vi "ColorScores.vi"() -> ()   [LabVIEW 2022 SP3]
uses:
  <vilib>/Utility/file.llb/Read Delimited Spreadsheet (DBL).vi
  <vilib>/Analysis/NI_AALBase.lvlib
panel:
  out "Array Constant":u8[](array[numeric])
  out "min score":sgl
  out "max score":sgl
  in  "Save to BMP":bool
  in  "Listbox":i32[](listbox)=[0]
  in  "Use Selected Files":bool
  in  "Color Table":u32[](array[colorbox])=[0, 0, 65793, 131586, 197379, 263172, 328965, 394758, 460551, 526344, 592137, 657930, 723723, 789516, 855309, 921102, 986895, 1052688, 1118481, 1184274, 1250067, 1315860, 1381653, 1447446, 1513239, 1579032, 1644825, 1710618, 1776411, 1842204, 1907997, 1973790, 2039583, 2105376, 2171169, 2236962, 2302755, 2368548, 2434341, 2500134, 2565927, 2631720, 2697513, 2763306, 2829099, 2894892, 2960685, 3026478, 3092271, 3158064, 3223857, 3289650, 3355443, 3421236, 3487029, 3552822, 3618615, 3684408, 3750201, 3815994, 3881787, 3947580, 4013373, 4079166, 4144959, 4210752, 4276545, 4342338, 4408131, 4473924, 4539717, 4605510, 4671303, 4737096, 4802889, 4868682, 4934475, 5000268, 5066061, 5131854, 5197647, 5263440, 5329233, 5395026, 5460819, 5526612, 5592405, 5658198, 5723991, 5789784, 5855577, 5921370, 5987163, 6052956, 6118749, 6184542, 6250335, 6316128, 6381921, 6447714, 6513507, 6579300, 6645093, 6710886, 6776679, 6842472, 6908265, 6974058, 7039851, 7105644, 7171437, 7237230, 7303023, 7368816, 7434609, 7500402, 7566195, 7631988, 7697781, 7763574, 7829367, 7895160, 7960953, 8026746, 8092539, 8158332, 8224125, 8289918, 8355711, 8421504, 8487297, 8553090, 8618883, 8684676, 8750469, 8816262, 8882055, 8947848, 9013641, 9079434, 9145227, 9211020, 9276813, 9342606, 9408399, 9474192, 9539985, 9605778, 9671571, 9737364, 9803157, 9868950, 9934743, 10000536, 10066329, 10132122, 10197915, 10263708, 10329501, 10395294, 10461087, 10526880, 10592673, 10658466, 10724259, 10790052, 10855845, 10921638, 10987431, 11053224, 11119017, 11184810, 11250603, 11316396, 11382189, 11447982, 11513775, 11579568, 11645361, 11711154, 11776947, 11842740, 11908533, 11974326, 12040119, 12105912, 12171705, 12237498, 12303291, 12369084, 12434877, 12500670, 12566463, 12632256, 12698049, 12763842, 12829635, 12895428, 12961221, 13027014, 13092807, 13158600, 13224393, 13290186, 13355979, 13421772, 13487565, 13553358, 13619151, 13684944, 13750737, 13816530, 13882323, 13948116, 14013909, 14079702, 14145495, 14211288, 14277081, 14342874, 14408667, 14474460, 14540253, 14606046, 14671839, 14737632, 14803425, 14869218, 14935011, 15000804, 15066597, 15132390, 15198183, 15263976, 15329769, 15395562, 15461355, 15527148, 15592941, 15658734, 15724527, 15790320, 15856113, 15921906, 15987699, 16053492, 16119285, 16185078, 16250871, 16316664, 16382457, 6352640, 12058434, 16770066, 16758546, 16711731]
  out "raw scores":dbl[][](graph)
  out "score coded":dbl[][](graph)
  in  "lookuptable":path=path "E:/junk/EYEFiles/99lktbl10-31.txt"
  out "intercept":u8[][](graph)
  out "midband":u8[][](graph)
  in  "thresholds":T1={"T1"=5.0, "T2"=6.0, "T3"=6.5, "T4"=7.0, "T5"=8.0} {"T5" format="%.2f"; "T4" format="%.2f"; "T3" format="%.2f"; "T2" format="%.2f"; "T1" format="%.2f"}
  in  "psa":dbl format="%.2f"
  in  "Range Params":T2={"mb max"=-20.0, "mb min"=-70.0, "slope max"=8.0, "slope min"=-8.0, "int max"=5.0, "int min"=-85.0} {"int min" format="%.2f"; "int max" format="%.2f"; "slope min" format="%.2f"; "slope max" format="%.2f"; "mb min" format="%.2f"; "mb max" format="%.2f"}
  in  "pixels in x":i32=256
  in  "pixels in y":i32=240
  in  "select directory with eye files":path
  # "T5 is highest threshold. Leave unused thresholds the same value as lowest valid threshold"
  # "color coded BMPs are saved for MBF and the score. The raw score image is also saved to BMP"
  # "Values for parameter images"
  # "Old B&K data often 346x240"
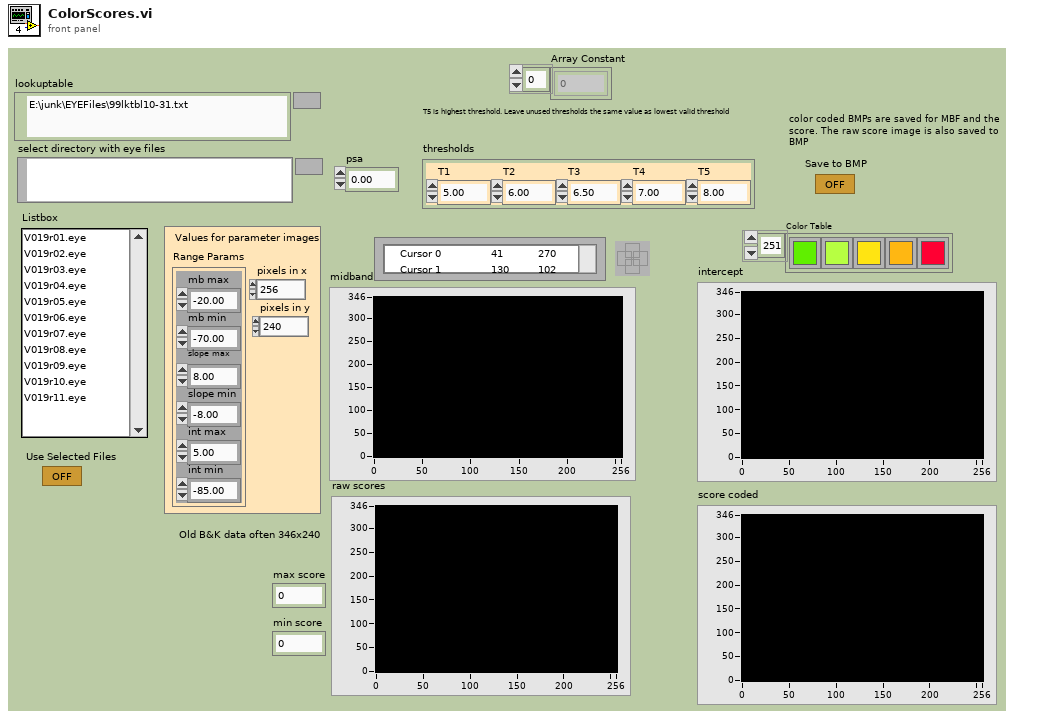
[diagram p1: front panel]
types:
  T1 = cluster{"T1":dbl, "T2":dbl, "T3":dbl, "T4":dbl, "T5":dbl}
  T2 = cluster{"mb max":dbl, "mb min":dbl, "slope max":dbl, "slope min":dbl, "int max":dbl, "int min":dbl}
  T3 = cluster{"[0]":dbl, "[1]":dbl, "[2]":dbl, "[3]":dbl, "[4]":dbl, "[5]":dbl, "[6]":dbl, "[7]":dbl}
  T4 = cluster{"[5]":dbl, "[4]":dbl, "[1]":dbl, "[0]":dbl, "[3]":dbl, "[2]":dbl}
  T5 = cluster{"Array Constant":u8[][], "Array Constant":u8[][], "Array Constant":u8[][]}
  T6 = cluster{"left":i16, "top":i16, "right":i16, "bottom":i16}
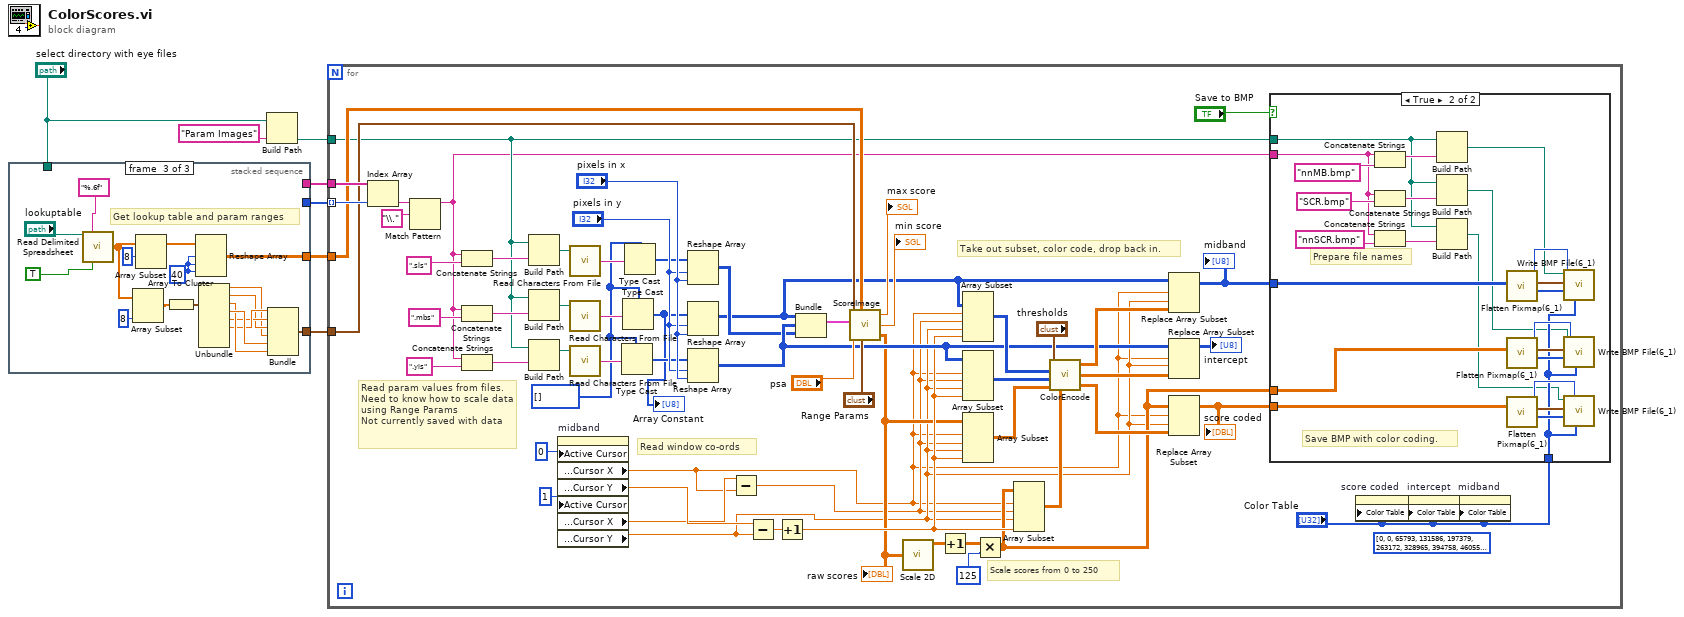
[diagram p0: block diagram]
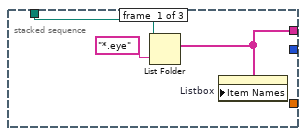
[diagram p3: hidden frame]
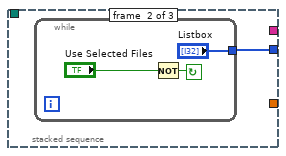
[diagram p4: hidden frame]
diagram:
  n1 = stacked-sequence {
    tunnel: [w9 _ _] -> w7
    tunnel: "select directory with eye files" -> [w8 _ _]
    tunnel: [_ w11 _] -> w6
    tunnel: [_ _ w17] -> w5
    tunnel: [_ _ w16] -> w4
    frame #0 {
      n2 = List Folder(path=w8, pattern="*.eye") -> (filenames=w9:string[])  [unwired: 1 in, 4 out]
      n3 = property on="Listbox" class="LstBox (strict)"("Item Names"=w9) -> ()  [unwired: 2 in, 2 out]
    }
    frame #1 {
      n4 = while {
        tunnel: ["Listbox"] -> w11
        stop <- w12 continue-if-true
        n5 = Not(x="Use Selected Files") -> (.not. x?=w12:bool)
      }
    }
    frame #2 {
      w20 = 40
      # "Get lookup table and param ranges"
      n6 = call-poly <vilib>:"Read Delimited Spreadsheet.vi"("file path (dialog if empty)"="lookuptable", "format (%.3f)"="%.6f", "transpose? (F)"=TRUE) -> ("first row"=w21:dbl[])  [unwired: 7 in, 5 out]
      n7 = Array Subset(array=w21, length=8) -> (w23:dbl[])  [unwired: 1 in]
      n8 = Array Subset(array=w21, index=8) -> (w19:dbl[])  [unwired: 1 in]
      n9 = Array To Cluster(array=w23) -> (cluster=w24:T3)
      n10 = Reshape Array(w19, w20, w20, w20) -> (w17:dbl[][][])
      n11 = Unbundle(w24) -> ("[0]"=w25:dbl, "[1]"=w26:dbl, "[2]"=w29:dbl, "[3]"=w30:dbl, "[4]"=w27:dbl, "[5]"=w28:dbl)  [unwired: 2 out]
      n12 = Bundle("[5]"=w28, "[4]"=w27, "[1]"=w26, "[0]"=w25, "[3]"=w30, "[2]"=w29) -> (w16:T4)  [unwired: 1 out]
    }
  }
  n13 = Build Path(base path="select directory with eye files", name or relative path="Param Images") -> (appended path=w1:path)
  n14 = for {
    tunnel: w7 -> [w75]
    tunnel: w6 -> [w74] mode=indexing
    tunnel: w5 -> [w66]
    tunnel: w4 -> [w65]
    tunnel: w1 -> [w41]
    w34 = u8[] [] ("Array Constant")
    (unwired) u32[] [0, 0, 65793, 131586, 197379, 263172, 328965, 394758, 460551, 526344, 592137, 657930, 723723, 789516, 855309, 921102, 986895, 1052688, 1118481, 1184274, 1250067, 1315860, 1381653, 1447446, 1513239, 1579032, 1644825, 1710618, 1776411, 1842204, 1907997, 1973790, 2039583, 2105376, 2171169, 2236962, 2302755, 2368548, 2434341, 2500134, 2565927, 2631720, 2697513, 2763306, 2829099, 2894892, 2960685, 3026478, 3092271, 3158064, 3223857, 3289650, 3355443, 3421236, 3487029, 3552822, 3618615, 3684408, 3750201, 3815994, 3881787, 3947580, 4013373, 4079166, 4144959, 4210752, 4276545, 4342338, 4408131, 4473924, 4539717, 4605510, 4671303, 4737096, 4802889, 4868682, 4934475, 5000268, 5066061, 5131854, 5197647, 5263440, 5329233, 5395026, 5460819, 5526612, 5592405, 5658198, 5723991, 5789784, 5855577, 5921370, 5987163, 6052956, 6118749, 6184542, 6250335, 6316128, 6381921, 6447714, 6513507, 6579300, 6645093, 6710886, 6776679, 6842472, 6908265, 6974058, 7039851, 7105644, 7171437, 7237230, 7303023, 7368816, 7434609, 7500402, 7566195, 7631988, 7697781, 7763574, 7829367, 7895160, 7960953, 8026746, 8092539, 8158332, 8224125, 8289918, 8355711, 8421504, 8487297, 8553090, 8618883, 8684676, 8750469, 8816262, 8882055, 8947848, 9013641, 9079434, 9145227, 9211020, 9276813, 9342606, 9408399, 9474192, 9539985, 9605778, 9671571, 9737364, 9803157, 9868950, 9934743, 10000536, 10066329, 10132122, 10197915, 10263708, 10329501, 10395294, 10461087, 10526880, 10592673, 10658466, 10724259, 10790052, 10855845, 10921638, 10987431, 11053224, 11119017, 11184810, 11250603, 11316396, 11382189, 11447982, 11513775, 11579568, 11645361, 11711154, 11776947, 11842740, 11908533, 11974326, 12040119, 12105912, 12171705, 12237498, 12303291, 12369084, 12434877, 12500670, 12566463, 12632256, 12698049, 12763842, 12829635, 12895428, 12961221, 13027014, 13092807, 13158600, 13224393, 13290186, 13355979, 13421772, 13487565, 13553358, 13619151, 13684944, 13750737, 13816530, 13882323, 13948116, 14013909, 14079702, 14145495, 14211288, 14277081, 14342874, 14408667, 14474460, 14540253, 14606046, 14671839, 14737632, 14803425, 14869218, 14935011, 15000804, 15066597, 15132390, 15198183, 15263976, 15329769, 15395562, 15461355, 15527148, 15592941, 15658734, 15724527, 15790320, 15856113, 15921906, 15987699, 16053492, 16119285, 16185078, 16250871, 16316664, 16382457, 6352640, 12058434, 16770066, 16758546, 16711731] ("Color Table")
    # "Read window co-ords"
    # "Read param values from files.\nNeed to know how to scale data using Range Params\nNot currently saved with data"
    # "Scale scores from 0 to 250"
    # "Take out subset, color code, drop back in."
    n15 = Index Array(array=w75, index=w74) -> (element=w47:string)
    n16 = Match Pattern(string=w47, regular expression="\\." ("search char (-)")) -> (before substring=w40:string)  [unwired: 4 out]
    n17 = Concatenate Strings(w40, ".sls") -> (w51:string)
    n18 = Concatenate Strings(w40, ".mbs") -> (w52:string)
    n19 = Concatenate Strings(w40, ".yis") -> (w53:string)
    n20 = Build Path(base path=w41, name or relative path=w51) -> (appended path=w60:path)
    n21 = Build Path(base path=w41, name or relative path=w52) -> (appended path=w61:path)
    n22 = Build Path(base path=w41, name or relative path=w53) -> (appended path=w62:path)
    n23 = property on="midband" class="IntGraph (strict)"("Active Cursor"=0, "Active Cursor"=1) -> ("Cursor.Cursor Position:Cursor X"=w37:dbl, "Cursor.Cursor Position:Cursor Y"=w43:dbl, "Cursor.Cursor Position:Cursor X"=w42:dbl, "Cursor.Cursor Position:Cursor Y"=w39:dbl)  [unwired: 2 in, 2 out]
    n24 = call <vilib>:"Read Characters From File.vi"("file path (dialog if empty)"=w60) -> ("character string"=w55:string)  [unwired: 1 in, 7 out]
    n25 = call <vilib>:"Read Characters From File.vi"("file path (dialog if empty)"=w61) -> ("character string"=w57:string)  [unwired: 1 in, 7 out]
    n26 = call <vilib>:"Read Characters From File.vi"("file path (dialog if empty)"=w62) -> ("character string"=w58:string)  [unwired: 1 in, 7 out]
    n27 = Type Cast(type=w34, x=w58) -> (*(type *) &x=w59:u8[])
    n28 = Type Cast(type=w34, x=w57) -> (*(type *) &x=w33:u8[])
    "Array Constant" <- w33
    n29 = Type Cast(type=w34, x=w55) -> (*(type *) &x=w56:u8[])
    n30 = Reshape Array(w56, "pixels in y", "pixels in x") -> (w36:u8[][])
    n31 = Reshape Array(w33, "pixels in y", "pixels in x") -> (w35:u8[][])
    n32 = Reshape Array(w59, "pixels in y", "pixels in x") -> (w78:u8[][])
    n33 = Subtract(x=w42, y=w37) -> (x-y=w38:dbl)
    n34 = Subtract(x=w43, y=w39) -> (x-y=w46:dbl)
    n35 = Increment(x=w46) -> (x+1=w72:dbl)
    n36 = Bundle("Array Constant"=w35, "Array Constant"=w78, "Array Constant"=w36) -> (w92:T5)  [unwired: 1 out]
    n37 = call "ScoreImage.vi"("Range Params LUTable"=w65, "LookUp Table"=w66, "fit data"=w92, "psa"="psa", "Range Params"="Range Params") -> ("max score"=→"max score":sgl, "min score"=→"min score":sgl, "score"=w71:dbl[][])  [unwired: 1 in]
    "raw scores" <- w71
    n38 = call <vilib>:"Scale 2D.vi"("X"=w71) -> ("Y=(X-offset)/scale"=w83:dbl[][])  [unwired: 3 out]
    n39 = Increment(x=w83) -> (x+1=w82:dbl[][])
    n40 = Array Subset(array=w35, index (row)=w37, length (row)=w38, index (col)=w39, length (col)=w72) -> (w84:u8[][])
    n41 = Array Subset(array=w78, index (row)=w37, length (row)=w38, index (col)=w39, length (col)=w72) -> (w85:u8[][])
    n42 = Array Subset(array=w71, index (row)=w37, length (row)=w38, index (col)=w39, length (col)=w72) -> (w86:dbl[][])
    n43 = Multiply(x=w82, y=125) -> (x*y=w69:dbl[][])
    n44 = Array Subset(array=w69, index (row)=w37, length (row)=w38, index (col)=w39, length (col)=w72) -> (w70:dbl[][])
    n45 = call "ColorEncode.vi"("thresholds"="thresholds", "midband in"=w84, "intercept in"=w85, "score in"=w86, "scaled score"=w70) -> ("midband out"=w88:dbl[][], "intercept out"=w89:dbl[][], "scaled score out"=w87:dbl[][])
    n46 = Replace Array Subset(array=w35, new element=w88, index (row)=w37, index (col)=w39) -> (w80:u8[][])
    "midband" <- w80
    n47 = Replace Array Subset(array=w78, new element=w89, index (row)=w37, index (col)=w39) -> (→"intercept":u8[][])
    n48 = Replace Array Subset(array=w69, new element=w87, index (row)=w37, index (col)=w39) -> (w79:dbl[][])
    "score coded" <- w79
    n49 = case shown="True" "Save to BMP" {
      tunnel: w80 -> [_ w108]
      tunnel: w69 -> [_ w107]
      tunnel: w79 -> [_ w106]
      tunnel: "Color Table" -> [_ w105]
      tunnel: w41 -> [_ w95]
      tunnel: w40 -> [_ w94]
      frame False {
      }
      frame True {
        # "Prepare file names"
        # "Save BMP with color coding."
        n50 = Concatenate Strings(w94, "nnMB.bmp") -> (w101:string)
        n51 = Concatenate Strings(w94, "SCR.bmp") -> (w100:string)
        n52 = Concatenate Strings(w94, "nnSCR.bmp") -> (w99:string)
        n53 = Build Path(base path=w95, name or relative path=w101) -> (appended path=w98:path)
        n54 = Build Path(base path=w95, name or relative path=w100) -> (appended path=w97:path)
        n55 = Build Path(base path=w95, name or relative path=w99) -> (appended path=w96:path)
        n56 = call <vilib>:"Flatten Pixmap(6_1).vi"("8-bit pixmap"=w108) -> ("flattened image data"=w116:u8[], "bounds"=w117:T6, "bit depth"=w115:u8)  [unwired: 3 in, 5 out]
        n57 = call <vilib>:"Flatten Pixmap(6_1).vi"("8-bit pixmap"=w107) -> ("flattened image data"=w113:u8[], "bounds"=w114:T6, "bit depth"=w112:u8)  [unwired: 3 in, 5 out]
        n58 = call <vilib>:"Flatten Pixmap(6_1).vi"("8-bit pixmap"=w106) -> ("flattened image data"=w110:u8[], "bounds"=w111:T6, "bit depth"=w109:u8)  [unwired: 3 in, 5 out]
        n59 = call <vilib>:"Write BMP File(6_1).vi"("color table"=w105, "depth"=w115, "flattened image data"=w116, "rect"=w117, "path to BMP file"=w98) -> ()  [unwired: 1 in, 6 out]
        n60 = call <vilib>:"Write BMP File(6_1).vi"("color table"=w105, "depth"=w112, "flattened image data"=w113, "rect"=w114, "path to BMP file"=w97) -> ()  [unwired: 1 in, 6 out]
        n61 = call <vilib>:"Write BMP File(6_1).vi"("color table"=w105, "depth"=w109, "flattened image data"=w110, "rect"=w111, "path to BMP file"=w96) -> ()  [unwired: 1 in, 6 out]
      }
    }
    n62 = property on="score coded" class="IntGraph (strict)"("Color Table"="Color Table") -> ()  [unwired: 2 in, 2 out]
    n63 = property on="intercept" class="IntGraph (strict)"("Color Table"="Color Table") -> ()  [unwired: 2 in, 2 out]
    n64 = property on="midband" class="IntGraph (strict)"("Color Table"="Color Table") -> ()  [unwired: 2 in, 2 out]
  }
